vi "ma_FFT Power Spectrum and PS Density no State (CDB).vi"(0 "time signal":waveform(cdb), 1 "restart averaging (F)":bool, 2 "ps density":bool, 5 "window":T1=1 items=["Rectangle"=0, "Hanning"=1, "Hamming"=2, "Blackman-Harris"=3, "Exact Blackman"=4, "Blackman"=5, "Flat Top"=6, "4 Term B-Harris "=7, "7 Term B-Harris"=8, "Low Sidelobe"=9, "Blackman Nuttall"=11, "Triangle"=30, "Bartlett-Hanning"=31, "Bohman"=32, "Parzen"=33, "Welch"=34, "Kaiser"=60, "Dolph-Chebyshev"=61, "Gaussian"=62], 7 "averaging parameters":T3={"averaging mode"=enum."No averaging", "weighting mode"=enum."Exponential", "number of averages"=10} {"number of averages" min=1}, 9 "dB On (F)":bool, 11 "error in":errorcluster, 12 "state info":T2 {"real spectrum" format="%0.2f"; "averages completed" format="%0.2f"; "df" format="%0.2f"; "complex spectrum" format="%0.2f"; "spectrum parameters"."window" items=["Rectangle"=0, "Hanning"=1, "Hamming"=2, "Blackman-Harris"=3, "Exact Blackman"=4, "Blackman"=5, "Flat Top"=6, "4 Term B-Harris "=7, "7 Term B-Harris"=8, "Low Sidelobe"=9, "Blackman Nuttall"=11, "Triangle"=30, "Bartlett-Hanning"=31, "Bohman"=32, "Parzen"=33, "Welch"=34, "Kaiser"=60, "Dolph-Chebyshev"=61, "Gaussian"=62]; "dt" format="%0.2f"; "timestamp" format="%0.2f"; "dt history" format="%0.2f"; "t0 history" format="%0.2f"}, 13 "window parameter":dbl=nan) -> (3 "averaging done":bool, 4 "power spectrum":cluster{"f0":dbl, "df":dbl, "magnitude":dbl[]} {"f0" format="%0.2p"; "df" format="%0.2p"; "magnitude" format="%0.2p"}, 10 "averages completed":dbl format="%0.2f", 14 "state info":T2 {"real spectrum" format="%0.2f"; "averages completed" format="%0.2f"; "df" format="%0.2f"; "complex spectrum" format="%0.2f"; "spectrum parameters"."window" items=["Rectangle"=0, "Hanning"=1, "Hamming"=2, "Blackman-Harris"=3, "Exact Blackman"=4, "Blackman"=5, "Flat Top"=6, "4 Term B-Harris "=7, "7 Term B-Harris"=8, "Low Sidelobe"=9, "Blackman Nuttall"=11, "Triangle"=30, "Bartlett-Hanning"=31, "Bohman"=32, "Parzen"=33, "Welch"=34, "Kaiser"=60, "Dolph-Chebyshev"=61, "Gaussian"=62]; "dt" format="%0.2f"; "timestamp" format="%0.2f"; "dt history" format="%0.2f"; "t0 history" format="%0.2f"}, 15 "error out":errorcluster)   [LabVIEW 2020, in "NI_MAPro.lvlib"]
doc: "Computes the averaged auto power spectrum of the input signal. Each time waveform corresponds to a single FFT block and has to be passed individually to this VI. Averaging parameters specifies how the averaging is performed. This includes the averaging mode (No averaging, vector averaging, RMS averaging, or peak hold), the weighting mode (linear or exponential), and the number of averages. Averages completed returns the number of averages completed so far."
uses:
  NI_MAPro.lvlib
  windowTd.ctl
  NI_MABase.lvlib
  NI_AALPro.lvlib
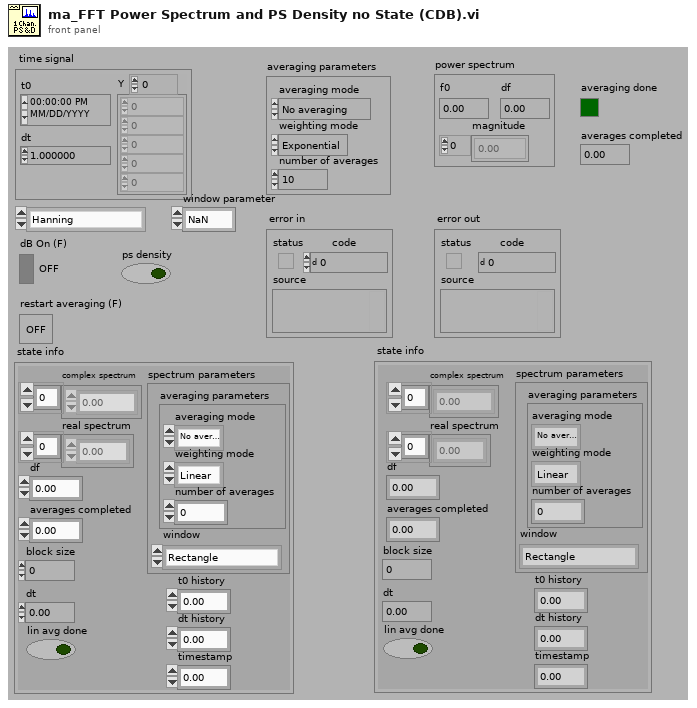
[diagram p1: front panel]
types:
  T1 = typedef "NI_AALPro.lvlib/windowTd.ctl" = u32
  T2 = cluster{"block size":i32, "dt":dbl, "spectrum parameters":cluster{"averaging parameters":cluster{"averaging mode":enum16{"No averaging", "Vector averaging", "RMS averaging", "Peak hold"}, "weighting mode":enum16{"Linear", "Exponential"}, "number of averages":u32}, "window":T1}, "df":dbl, "averages completed":dbl, "complex spectrum":cdb[], "real spectrum":dbl[], "t0 history":dbl, "dt history":dbl, "timestamp":dbl, "lin avg done":bool}
  T3 = cluster{"averaging mode":enum16{"No averaging", "Vector averaging", "RMS averaging", "Peak hold"}, "weighting mode":enum16{"Linear", "Exponential"}, "number of averages":u32}
  T4 = enum16{"FFT spectrum", "Power spectrum", "Cross spectrum", "Frequency response"}
  T5 = enum16{"No averaging", "Vector averaging", "RMS averaging", "Peak hold"}
  T6 = cluster{"f0":dbl, "df":dbl, "spectrum in dB":dbl[]}
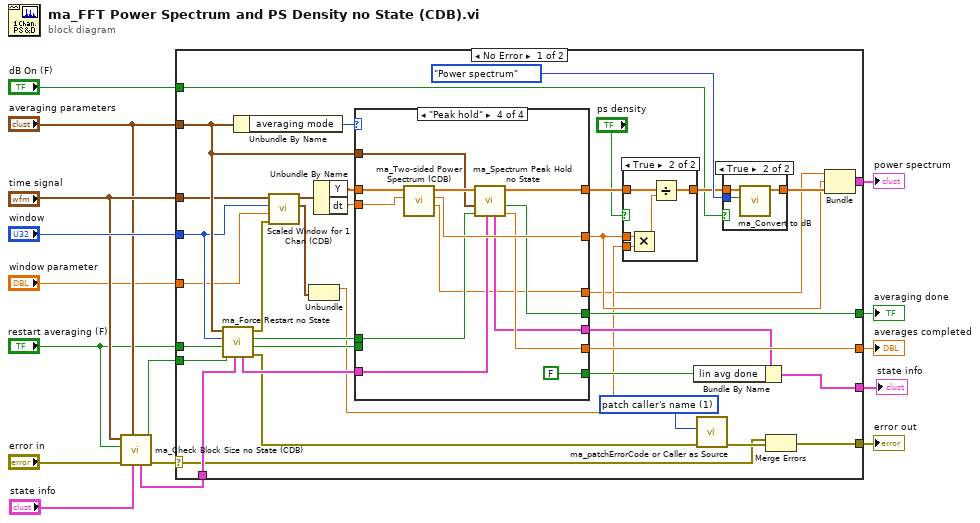
[diagram p0: block diagram]
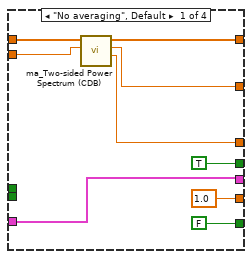
[diagram p3: hidden frame]
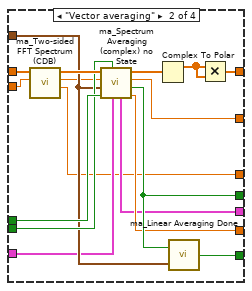
[diagram p4: hidden frame]
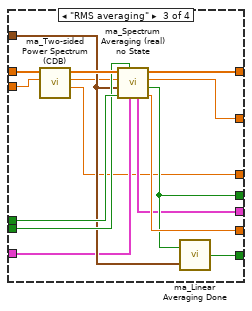
[diagram p5: hidden frame]
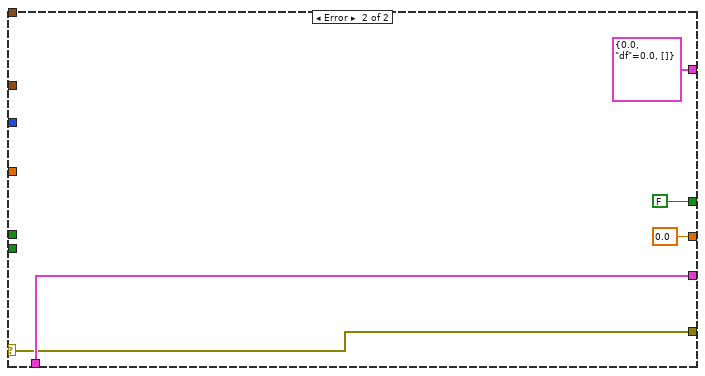
[diagram p7: hidden frame]
diagram:
  n1 = call "ma_Check Block Size no State (CDB).vi"("state info"="state info", "averaging parameters"="averaging parameters", "error in"="error in", "restart averaging (F)"="restart averaging (F)", "time signal"="time signal") -> ("error out"=w3:errorcluster, "force restart averaging"=w4:bool, "state info"=w6:T2)  [unwired: 1 in, 3 out]
  n2 = case shown="No Error" w3 {
    selector: w3 -> [w17 w117]
    tunnel: "averaging parameters" -> [w52 _]
    tunnel: [w51 0.0] -> w16
    tunnel: "window" -> [w50 _]
    tunnel: [w48 FALSE ("averaging done")] -> w14
    tunnel: "time signal" -> [w47 _]
    tunnel: "restart averaging (F)" -> [w46 _]
    tunnel: [w20 w117] -> w12
    tunnel: "dB On (F)" -> [w25 _]
    tunnel: [w44 cluster{dbl, "df":dbl, dbl[]} {0.0, "df"=0.0, []}] -> w8
    tunnel: w6 -> [w33 w118]
    tunnel: [w42 w118] -> w5
    tunnel: w4 -> [w26 _]
    tunnel: "window parameter" -> [w21 _]
    frame No Error {
      w23 = u16 1 items=["patch error code", "patch caller's name"] ("operation")
      n3 = call "ma_Force Restart no State.vi"("state info"=w33, "force restart averaging in"=w26, "restart averaging (F)"=w46, "window"=w50, "averaging parameters"=w52) -> ("error out"=w18:errorcluster, "retrieve last spectrum"=w35:bool, "force restart averaging"=w36:bool, "skip processing"=w37:errorcluster, "state info"=w34:T2)  [unwired: 1 in, 1 out]
      n4 = Unbundle By Name(w52) -> ("averaging mode"=w41:T5)
      n5 = call "Scaled Window for 1 Chan (CDB).vi"("error in (no error)"=w37, "window parameter"=w21, "window"=w50, "signal in"=w47) -> ("window constants"=w31:cluster{"eq noise BW":dbl, "coherent gain":dbl}, "signal out"=w38:waveform(cdb))  [unwired: 5 in, 1 out]
      n6 = Unbundle(w31) -> ("eq noise BW"=w24:dbl)  [unwired: 1 out]
      n7 = Unbundle By Name(w38) -> ("Y"=w39:cdb[], "dt"=w40:dbl)
      n8 = case shown="\"Peak hold\"" w41 {
        tunnel: w39 -> [w66 w80 w97 w112]
        tunnel: [w64 w73 w91 w110] -> w28
        tunnel: [w63 w81 w98 w107] -> w30
        tunnel: w52 -> [_ w75 w92 w103]
        tunnel: w36 -> [_ w84 w99 w108]
        tunnel: [1.0 ("averages completed") w71 w89 w106] -> w51
        tunnel: w40 -> [w65 w79 w96 w111]
        tunnel: [TRUE ("averaging done") w72 w88 w104] -> w48
        tunnel: [FALSE w77 w94 FALSE] -> w43
        tunnel: w35 -> [_ w76 w93 _]
        tunnel: w34 -> [w60 w70 w87 w102]
        tunnel: [w60 w69 w86 w101] -> w32
        tunnel: [w59 w68 w85 w100] -> w22
        frame "No averaging", Default {
          n9 = call "ma_Two-sided Power Spectrum (CDB).vi"("dt"=w65, "signal (V)"=w66) -> ("f0"=w59:dbl, "df"=w64:dbl, "power spectrum (V^2 rms)"=w63:dbl[])  [unwired: 1 in, 6 out]
        }
        frame "Vector averaging" {
          n10 = call "ma_Two-sided FFT Spectrum (CDB).vi"("dt"=w79, "signal (V)"=w80) -> ("f0"=w68:dbl, "df"=w74:dbl, "FFT spectrum (Vrms)"=w78:cdb[])  [unwired: 1 in, 6 out]
          n11 = call "ma_Spectrum Averaging (complex) no State.vi"("state info"=w70, "retrieve last spectrum (F)"=w76, "restart averaging (F)"=w84, "averaging parameters"=w75, "df"=w74, "complex spectrum"=w78) -> ("averages completed"=w71:dbl, "averaging done"=w72:bool, "df"=w73:dbl, "averaged complex spectrum"=w83:cdb[], "state info"=w69:T2)  [unwired: 1 out]
          n12 = Complex To Polar(r * e^(i*theta)=w83) -> (r=w82:dbl[])  [unwired: 1 out]
          n13 = call "ma_Linear Averaging Done.vi"("averaging parameters"=w75, "averaging done"=w72) -> ("linear averaging done"=w77:bool)
          n14 = Multiply(x=w82, y=w82) -> (x*y=w81:dbl[])
        }
        frame "RMS averaging" {
          n15 = call "ma_Two-sided Power Spectrum (CDB).vi"("dt"=w96, "signal (V)"=w97) -> ("f0"=w85:dbl, "df"=w90:dbl, "power spectrum (V^2 rms)"=w95:dbl[])  [unwired: 1 in, 6 out]
          n16 = call "ma_Spectrum Averaging (real) no State.vi"("state info"=w87, "retrieve last spectrum (F)"=w93, "restart averaging (F)"=w99, "averaging parameters"=w92, "df"=w90, "real spectrum"=w95) -> ("averages completed"=w89:dbl, "averaging done"=w88:bool, "df"=w91:dbl, "averaged real spectrum"=w98:dbl[], "state info"=w86:T2)  [unwired: 1 out]
          n17 = call "ma_Linear Averaging Done.vi"("averaging parameters"=w92, "averaging done"=w88) -> ("linear averaging done"=w94:bool)
        }
        frame "Peak hold" {
          n18 = call "ma_Two-sided Power Spectrum (CDB).vi"("dt"=w111, "signal (V)"=w112) -> ("f0"=w100:dbl, "df"=w110:dbl, "power spectrum (V^2 rms)"=w109:dbl[])  [unwired: 1 in, 6 out]
          n19 = call "ma_Spectrum Peak Hold no State.vi"("state info"=w102, "restart averaging (F)"=w108, "averaging parameters"=w103, "real spectrum"=w109) -> ("averages completed"=w106:dbl, "averaging done"=w104:bool, "peak spectrum"=w107:dbl[], "state info"=w101:T2)  [unwired: 4 out]
        }
      }
      n20 = case shown="True" "ps density" {
        tunnel: w30 -> [w53 w57]
        tunnel: [w53 w56] -> w29
        tunnel: w24 -> [_ w55]
        tunnel: w28 -> [_ w54]
        frame False {
        }
        frame True {
          n21 = Multiply(x=w54, y=w55) -> (x*y=w58:dbl)
          n22 = Divide(x=w57, y=w58) -> (x/y=w56:dbl[])
        }
      }
      n23 = Bundle By Name(cluster=w32, "lin avg done"=w43) -> (w42:T2)
      n24 = call "ma_patchErrorCode or Caller as Source.vi"("error in (no error)"=w18, "operation"=w23) -> ("error out"=w19:errorcluster)  [unwired: 2 in, 7 out]
      n25 = case shown="True" w25 {
        tunnel: w29 -> [w113 w116]
        tunnel: [w113 w115] -> w45
        tunnel: T4."Power spectrum" ("spectrum type") -> [_ w114]
        frame False {
        }
        frame True {
          n26 = call "ma_Convert to dB.vi"("spectrum type"=w114, "spectrum"=w116) -> ("spectrum in dB"=w115:dbl[])  [unwired: 9 out]
        }
      }
      n27 = Merge Errors(w17, w19) -> (w20:errorcluster)
      n28 = Bundle("f0"=w22, "df"=w28, "spectrum in dB"=w45) -> (w44:T6)  [unwired: 1 out]
    }
    frame Error {
    }
  }
  "averages completed" <- w16
  "error out" <- w12
  "averaging done" <- w14
  "power spectrum" <- w8
  "state info" <- w5
